vi "ALL.vi"   [LabVIEW 2011]
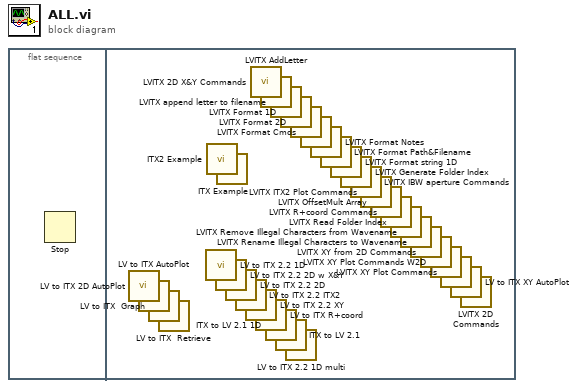
[diagram p0: block diagram]
diagram:
  n1 = flat-sequence {
    frame #0 {
      n2 = Stop() -> ()  [unwired: 1 in]
    }
    frame #1 {
      n3 = call "LV to ITX 2D AutoPlot.vi"() -> ()  [unwired: 15 in, 1 out]
      n4 = call "LV to ITX AutoPlot.vi"() -> ()  [unwired: 15 in, 1 out]
      n5 = call "LV to ITX  Graph.vi"() -> ()  [unwired: 12 in]
      n6 = call "LV to ITX  Retrieve.vi"() -> ()  [unwired: 11 in, 5 out]
      n7 = call "LV to ITX 2.2 1D.vi"() -> ()  [unwired: 12 in]
      n8 = call "ITX2 Example.vi"() -> ()  [unwired: 12 in]
      n9 = call "LV to ITX 2.2 2D w X&Y.vi"() -> ()  [unwired: 11 in, 1 out]
      n10 = call "ITX Example.vi"() -> ()  [unwired: 12 in]
      n11 = call "LV to ITX 2.2 2D.vi"() -> ()  [unwired: 12 in]
      n12 = call "LV to ITX 2.2 ITX2.vi"() -> ()  [unwired: 11 in, 1 out]
      n13 = call "LV to ITX 2.2 XY.vi"() -> ()  [unwired: 11 in, 1 out]
      n14 = call "LVITX 2D X&Y Commands.vi"() -> ()  [unwired: 4 in, 1 out]
      n15 = call "LV to ITX R+coord.vi"() -> ()  [unwired: 12 in]
      n16 = call "LVITX AddLetter.vi"() -> ()  [unwired: 1 in, 1 out]
      n17 = call "ITX to LV 2.1 1D.vi"() -> ()  [unwired: 3 in, 3 out]
      n18 = call "LVITX append letter to filename.vi"() -> ()  [unwired: 1 in, 1 out]
      n19 = call "ITX to LV 2.1.vi"() -> ()  [unwired: 2 in, 4 out]
      n20 = call "LVITX Format 1D.vi"() -> ()  [unwired: 2 in, 1 out]
      n21 = call "LV to ITX 2.2 1D multi.vi"() -> ()  [unwired: 12 in]
      n22 = call "LVITX Format 2D.vi"() -> ()  [unwired: 2 in, 1 out]
      n23 = call "LVITX Format Cmds.vi"() -> ()  [unwired: 1 in, 1 out]
      n24 = call "LVITX Format Notes.vi"() -> ()  [unwired: 1 in, 1 out]
      n25 = call "LVITX Format Path&Filename.vi"() -> ()  [unwired: 2 in, 2 out]
      n26 = call "LVITX Format string 1D.vi"() -> ()  [unwired: 2 in, 1 out]
      n27 = call "LVITX Generate Folder Index.vi"() -> ()  [unwired: 12 in]
      n28 = call "LVITX IBW aperture Commands.vi"() -> ()  [unwired: 4 in, 1 out]
      n29 = call "LVITX ITX2 Plot Commands.vi"() -> ()  [unwired: 6 in, 1 out]
      n30 = call "LVITX OffsetMult Array.vi"() -> ()  [unwired: 3 in, 1 out]
      n31 = call "LVITX R+coord Commands.vi"() -> ()  [unwired: 15 in, 1 out]
      n32 = call "LVITX Read Folder Index.vi"() -> ()  [unwired: 11 in, 1 out]
      n33 = call "LVITX Remove Illegal Characters from Wavename.vi"() -> ()  [unwired: 1 in, 1 out]
      n34 = call "LVITX Rename Illegal Characters to Wavename.vi"() -> ()  [unwired: 1 in, 1 out]
      n35 = call "LVITX XY from 2D Commands.vi"() -> ()  [unwired: 2 in, 1 out]
      n36 = call "LVITX XY Plot Commands W2D.vi"() -> ()  [unwired: 5 in, 1 out]
      n37 = call "LVITX XY Plot Commands.vi"() -> ()  [unwired: 6 in, 1 out]
      n38 = call "LV to ITX XY AutoPlot.vi"() -> ()  [unwired: 15 in, 1 out]
      n39 = call "LVITX 2D Commands.vi"() -> ()  [unwired: 15 in, 1 out]
    }
  }
